vi "Replace Item at Offset.vi"(8 "error in (no error)":errorcluster, 9 "New JSON Item":string, 10 "Offset of Item to Replace":i32, 11 "JSON":string) -> (0 "error out":errorcluster, 3 "<JSON>":string)   [LabVIEW 2017, in "JSONtext.lvlib"]
doc: "Replace the JSON Value located at an Offset in the input JSON. The Offset can be that returned by a previous \"Find\" operation on the input JSON."
uses:
  JSONtext.lvlib
  Parsing/Advance past whitespace.vi
  <vilib>/Utility/error.llb/Error Cluster From Error Code.vi
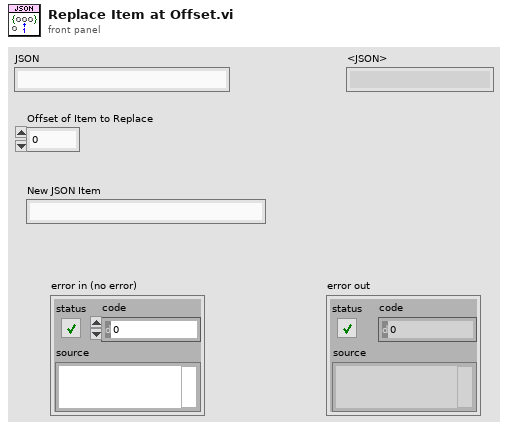
[diagram p1: front panel]
types:
  T1 = typedef "JSONtext.lvlib/Parsing State.ctl" = enum16{"Parser Error", "Object", "Array", "String", "Number/Other", "Leading Whitespace", "Object end", "Array end", "Value end"}
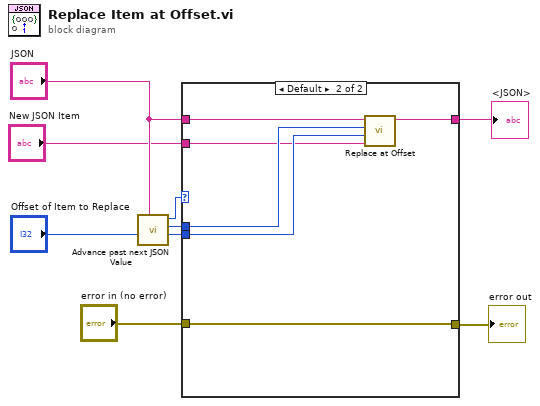
[diagram p0: block diagram]
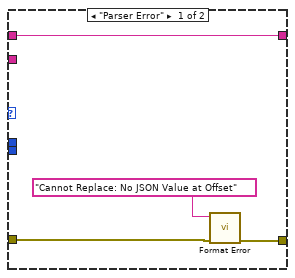
[diagram p2: hidden frame]
diagram:
  n1 = call "Advance past next JSON Value.vi"("JSON"="JSON", "Offset"="Offset of Item to Replace") -> ("Offset out"=w7:i32, "Value start"=w8:i32, "State"=w6:T1)  [unwired: 7 in]
  n2 = case shown="Default" w6 {
    tunnel: w8 -> [_ w19]
    tunnel: w7 -> [_ w18]
    tunnel: "JSON" -> [w13 w17]
    tunnel: [w13 w16] -> w4
    tunnel: "New JSON Item" -> [_ w15]
    tunnel: "error in (no error)" -> [w11 w14]
    tunnel: [w10 w14] -> w1
    frame "Parser Error" {
      n3 = call "Format Error.vi"("error in (no error)"=w11, "error message"="Cannot Replace: No JSON Value at Offset") -> ("error out"=w10:errorcluster)  [unwired: 9 in]
    }
    frame Default {
      n4 = call "Replace at Offset.vi"("JSON to Insert"=w15, "Offset past Item"=w18, "Item offset"=w19, "<JSON> in"=w17) -> ("<JSON>"=w16:string)  [unwired: 6 in, 1 out]
    }
  }
  "<JSON>" <- w4
  "error out" <- w1
